vi "PID.vi"   [LabVIEW 2020, in "NI_PID_pid.lvlib"]
doc: "Implements a PID controller using a PID algorithm for simple PID applications or high speed control applications that require an efficient algorithm. The PID algorithm features control output range limiting with integrator anti-windup and bumpless controller output for PID gain changes. Use the DBL instance of this VI to implement a single control loop. Use the DBL Array instance to implement parallel multi-loop control."
uses:
  <vilib>/addons/control/pid/NI_PID_pid.lvlib
  <vilib>/addons/control/pid/NI_PID__prctrl compat.lvlib
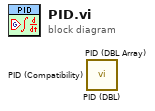
[diagram p0: block diagram]
diagram:
  n1 = call <vilib>:"PID (DBL).vi"() -> ()  [unwired: 10 in, 2 out]
  n2 = call <vilib>:"PID (DBL Array).vi"() -> ()  [unwired: 10 in, 2 out]
  n3 = call <vilib>:"PID (Compatibility).vi"() -> ()  [unwired: 11 in, 1 out]
